vi "AutoPush.vi"(0 "Simple push":dbl, 1 "PushActionMode":T1, 7 "LeftJoystick":dbl, 9 "RightJoystick":dbl, 12 "error in (no error)":errorcluster) -> (15 "error out":errorcluster)   [LabVIEW 2013]
uses:
  SingleSolenoidAction.ctl
  PushMode.ctl
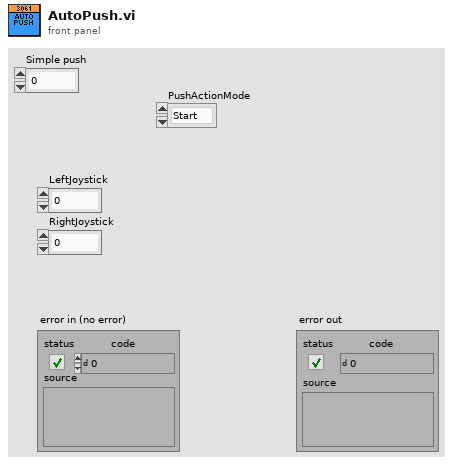
[diagram p1: front panel]
types:
  T1 = typedef "PushMode.ctl" = enum16{"Start", "Push", "Simple", "noAccelPush", "Stop"}
  T2 = typedef "SingleSolenoidAction.ctl" = enum16{"Init", "SetState", "Disable"}
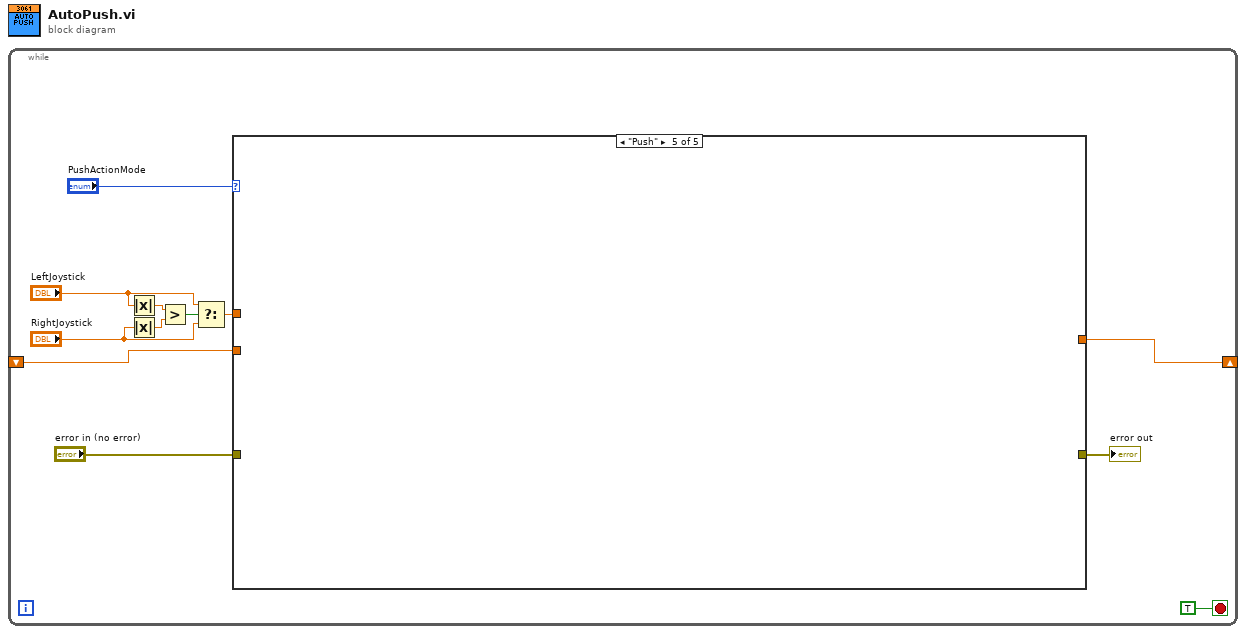
[diagram p0: block diagram]
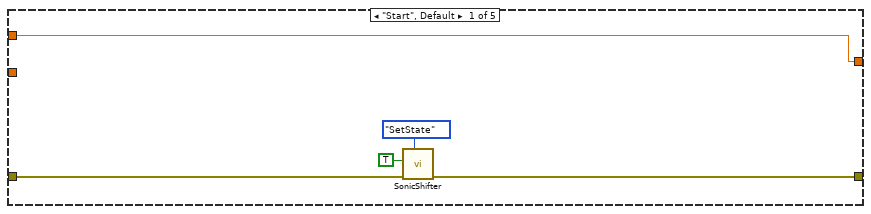
[diagram p2: hidden frame]
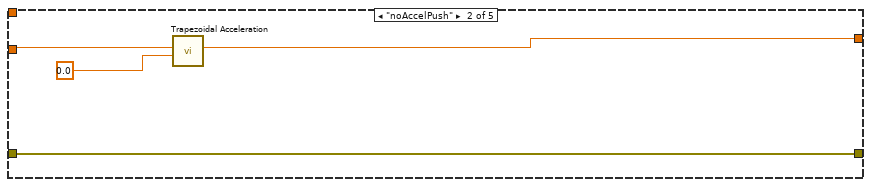
[diagram p3: hidden frame]
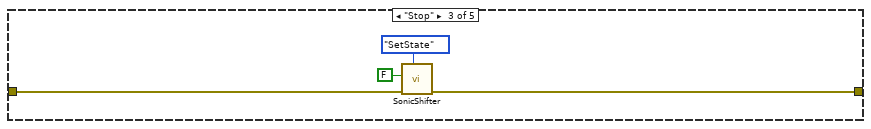
[diagram p4: hidden frame]
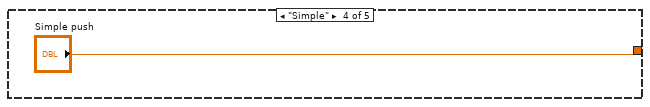
[diagram p5: hidden frame]
diagram:
  n1 = while {
    shift-right: [w2] -> _
    shift-left: _ -> [w1]
    stop <- TRUE stop-if-true
    n2 = Absolute Value(x="LeftJoystick") -> (abs(x)=w5:dbl)
    n3 = Absolute Value(x="RightJoystick") -> (abs(x)=w8:dbl)
    n4 = Greater?(x=w5, y=w8) -> (0:w4:bool)
    n5 = Select(t="LeftJoystick", s=w4, f="RightJoystick") -> (s? t:f=w3:dbl)
    n6 = case shown="\"Push\"" "PushActionMode" {
      tunnel: "error in (no error)" -> [w15 w21 w23 _ _]
      tunnel: [w14 w21 w22 _ _] -> w10
      tunnel: w3 -> [w13 _ _ _ _]
      tunnel: [w13 w20 _ "Simple push" _] -> w2
      tunnel: w1 -> [_ w19 _ _ _]
      frame "Start", Default {
        n7 = call "SonicShifter.vi"("Action"=SingleSolenoidAction."SetState", "error in (no error)"=w15, "Actuate?"=TRUE) -> ("error out"=w14:errorcluster)  [unwired: 8 in]
      }
      frame "noAccelPush" {
        n8 = call "Trapezoidal Acceleration.vi"("Desired"=0.0, "Actual"=w19) -> ("New Actual"=w20:dbl)  [unwired: 8 in, 1 out]
      }
      frame "Stop" {
        n9 = call "SonicShifter.vi"("Action"=SingleSolenoidAction."SetState", "error in (no error)"=w23, "Actuate?"=FALSE) -> ("error out"=w22:errorcluster)  [unwired: 8 in]
      }
      frame "Simple" {
      }
      frame "Push" {
      }
    }
    "error out" <- w10
  }
